vi "Destroy.vi"(10 "Self Event":refnum<data-value>) -> (0 "error out":errorcluster)   [LabVIEW 2021, in "jettl.lvlib" / "Self Event.lvlib"]
uses:
  Self Event.lvlib
  Msg Strategy/Msg Strategy.lvclass
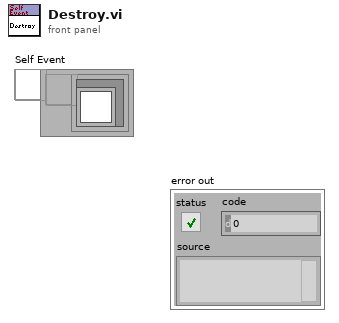
[diagram p1: front panel]
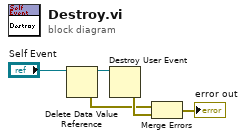
[diagram p0: block diagram]
diagram:
  n1 = Delete Data Value Reference(data value reference="Self Event") -> (data value=w5:refnum<user-event>, error out=w2:errorcluster)  [unwired: 1 in]
  n2 = Destroy User Event(user event=w5) -> (error out=w4:errorcluster)  [unwired: 1 in]
  n3 = Merge Errors(w2, w4) -> (→"error out":errorcluster)
